vi "Instrument Type ID.vi"() -> (1 "instrument type id":string="niDCPower")   [LabVIEW 2021, in "Session Management niDAQmx.lvlib"]
uses:
  Session Management niDAQmx.lvlib
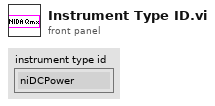
[diagram p1: front panel]
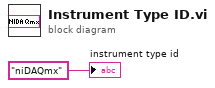
[diagram p0: block diagram]
diagram:
  "instrument type id" <- "niDAQmx"
